vi "SwerveCalculations.vi"(9 "j2x":dbl, 10 "j1y":dbl, 11 "j1x":dbl) -> (0 "magnitude4":dbl, 1 "magnitude3":dbl, 2 "magnitude2":dbl, 3 "magnitude1":dbl, 4 "Wheel Angle4":dbl, 5 "Wheel Angle2":dbl, 6 "Wheel Angle3":dbl, 7 "wheel angle 1":dbl)   [LabVIEW 2019]
panel:
  in  "width":dbl=26.0
  in  "length":dbl=26.0
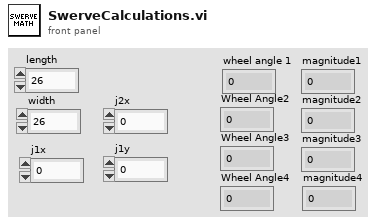
[diagram p1: front panel]
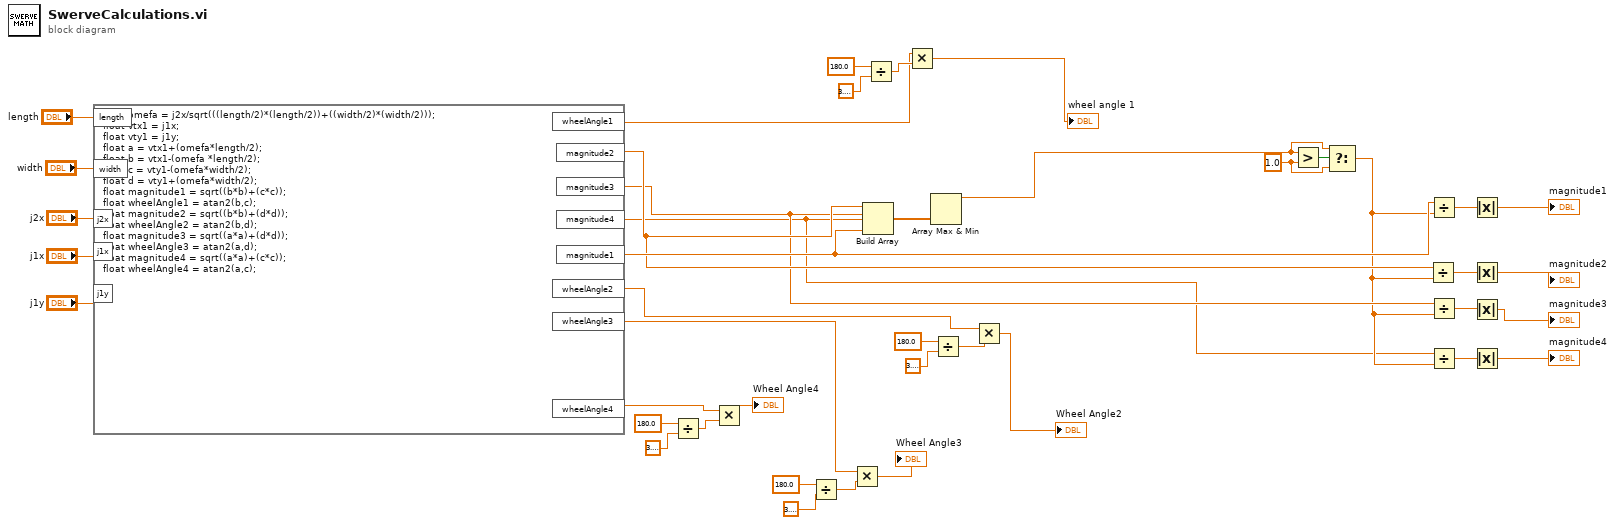
[diagram p0: block diagram]
diagram:
  w11 = 1.0 ("y")
  n1 = formula code="float omefa = j2x/sqrt(((length/2)*(length/2))+((width/2)*(width/2)));\nfloat vtx1 = j1x;\nfloat vty1 = j1y;\nfloat a = vtx1+(omefa*length/2);\nfloat b = vtx1-(omefa *length/2);\nfloat c = vty1-(omefa*width/2);\nfloat d = vty1+(omefa*width/2);\nfloat magnitude1 = sqrt((b*b)+(c*c));\nfloat wheelAngle1 = atan2(b,c);\nfloat magnitude2 = sqrt((b*b)+(d*d));\nfloat wheelAngle2 = atan2(b,d);\nfloat magnitude3 = sqrt((a*a)+(d*d));\nfloat wheelAngle3 = atan2(a,d);\nfloat magnitude4 = sqrt((a*a)+(c*c));\nfloat wheelAngle4 = atan2(a,c);"("length"="length", "width"="width", "j2x"="j2x", "j1y"="j1y", "j1x"="j1x") -> ("wheelAngle1"=w22:dbl, "magnitude1"=w9:dbl, "magnitude2"=w7:dbl, "magnitude3"=w5:dbl, "magnitude4"=w2:dbl, "wheelAngle2"=w18:dbl, "wheelAngle3"=w30:dbl, "wheelAngle4"=w33:dbl)
  n2 = Divide(x=180.0, y=3.141592653589793) -> (x/y=w34:dbl)
  n3 = Multiply(x=w33, y=w34) -> (x*y=→"Wheel Angle4":dbl)
  n4 = Divide(x=180.0, y=3.141592653589793) -> (x/y=w29:dbl)
  n5 = Multiply(x=w30, y=w29) -> (x*y=→"Wheel Angle3":dbl)
  n6 = Build Array(w7, w5, w2, w9) -> (w37:dbl[])
  n7 = Divide(x=180.0, y=3.141592653589793) -> (x/y=w23:dbl)
  n8 = Multiply(x=w22, y=w23) -> (x*y=→"wheel angle 1":dbl)
  n9 = Array Max & Min(array=w37) -> (max value=w10:dbl)  [unwired: 3 out]
  n10 = Divide(x=180.0, y=3.141592653589793) -> (x/y=w17:dbl)
  n11 = Multiply(x=w18, y=w17) -> (x*y=→"Wheel Angle2":dbl)
  n12 = Greater?(x=w10, y=w11) -> (0:w12:bool)
  n13 = Select(t=w10, s=w12, f=w11) -> (s? t:f=w3:dbl)
  n14 = Divide(x=w7, y=w3) -> (x/y=w6:dbl)
  n15 = Divide(x=w9, y=w3) -> (x/y=w8:dbl)
  n16 = Divide(x=w5, y=w3) -> (x/y=w4:dbl)
  n17 = Divide(x=w2, y=w3) -> (x/y=w1:dbl)
  n18 = Absolute Value(x=w8) -> (abs(x)=→"magnitude1":dbl)
  n19 = Absolute Value(x=w6) -> (abs(x)=→"magnitude2":dbl)
  n20 = Absolute Value(x=w4) -> (abs(x)=→"magnitude3":dbl)
  n21 = Absolute Value(x=w1) -> (abs(x)=→"magnitude4":dbl)
